vi "Cluster-typedefControls.vi"() -> ()   [LabVIEW 2016, in "test_ValueSignal.lvlib"]
uses:
  test_ValueSignal.lvlib
  main/apis/Stimulus/ValueSignalByPathString.vi
  main/apis/Assert/AssertControlValueByPathString.vi
  <vilib>/addons/_JKI Toolkits/Caraya/classes/Assert/Assert Equal Value and Type_Variant.vi
  <vilib>/addons/_JKI Toolkits/Caraya/classes/Test/Test.lvclass
  <vilib>/addons/_JKI Toolkits/Caraya/classes/Assert/Assert.lvclass
panel:
  out "error out":errorcluster
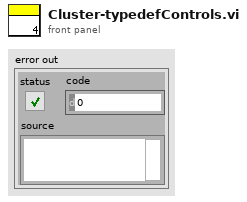
[diagram p1: front panel]
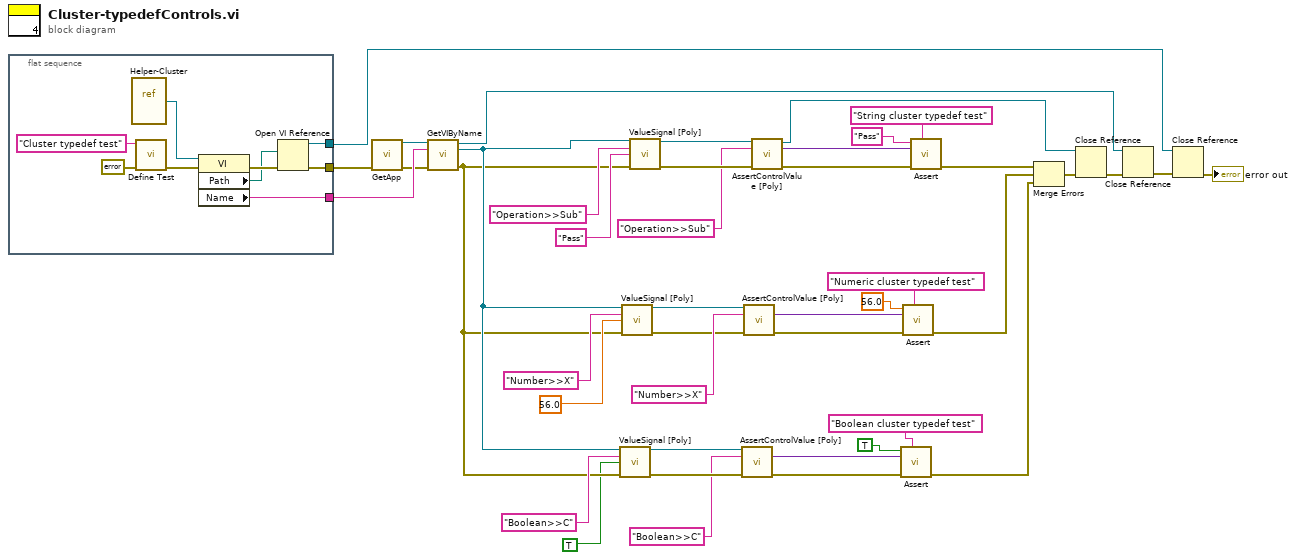
[diagram p0: block diagram]
diagram:
  n1 = flat-sequence {
    tunnel: [w48] -> w42
    tunnel: [w47] -> w27
    tunnel: [w45] -> w41
    frame #0 {
      n2 = vi-ref "Helper-Cluster.vi"() -> (w50:refnum<vi>)
      n3 = call <vilib>:"Define Test.vi"("error in (no error)"=errorcluster {"status"=FALSE, "code"=0, "source"=""}, "Label (VI Title)"="Cluster typedef test") -> ("error out"=w51:errorcluster)  [unwired: 9 in]
      n4 = property on="Property Node" class="VI"(reference=w50, error in=w51) -> (error out=w49:errorcluster, "Path"=w46:path, "Name"=w45:string)  [unwired: 1 out]
      n5 = Open VI Reference(vi path=w46, error in (no error)=w49) -> (vi reference=w47:refnum<vi>, error out=w48:errorcluster)  [unwired: 4 in]
    }
  }
  n6 = call "GetApp.vi"("error in (no error)"=w42) -> ("Application Ref"=w43:refnum<vi>, "error out"=w40:errorcluster)  [unwired: 13 in]
  n7 = call "GetVIByName.vi"("Application Ref in"=w43, "VI Name"=w41, "error in (no error)"=w40) -> ("Application Ref out"=w29:refnum<vi>, "VI Reference"=w5:refnum<vi>, "error out"=w4:errorcluster)  [unwired: 10 in]
  n8 = call-poly "ValueSignal [Poly].vi"("VI Reference In"=w5, "Control Name"="Boolean>>C", "Value (Signaling)"=TRUE, "error in"=w4) -> ("VI Reference Out"=w13:refnum<vi>, "error out"=w12:errorcluster)  [unwired: 10 in]
  n9 = call-poly "ValueSignal [Poly].vi"("VI Reference In"=w5, "Control Name"="Number>>X", "Value (Signaling)"=56.0, "error in"=w4) -> ("VI Reference Out"=w19:refnum<vi>, "error out"=w20:errorcluster)  [unwired: 10 in]
  n10 = call-poly "ValueSignal [Poly].vi"("VI Reference In"=w5, "Control Name"="Operation>>Sub", "Value (Signaling)"="Pass" ("Control Name"), "error in"=w4) -> ("VI Reference Out"=w39:refnum<vi>, "error out"=w38:errorcluster)  [unwired: 10 in]
  n11 = call-poly "AssertControlValue [Poly].vi"("VI Reference In"=w13, "Control Name"="Boolean>>C", "error in"=w12) -> ("Value"=w8:variant, "error out"=w9:errorcluster)  [unwired: 10 in, 1 out]
  n12 = call-poly "AssertControlValue [Poly].vi"("VI Reference In"=w19, "Control Name"="Number>>X", "error in"=w20) -> ("Value"=w24:variant, "error out"=w23:errorcluster)  [unwired: 10 in, 1 out]
  n13 = call-poly "AssertControlValue [Poly].vi"("VI Reference In"=w39, "Control Name"="Operation>>Sub", "error in"=w38) -> ("VI Reference Out"=w31:refnum<vi>, "Value"=w33:variant, "error out"=w34:errorcluster)  [unwired: 10 in]
  n14 = call-poly <vilib>:"Assert.vi"("Label"="Boolean cluster typedef test" ("Label (VI Title)"), "error in (no error)"=w9, "Y"=w8, "X"=TRUE) -> ("error out"=w6:errorcluster)  [unwired: 7 in]
  n15 = call-poly <vilib>:"Assert.vi"("Label"="Numeric cluster typedef test" ("Label (VI Title)"), "error in (no error)"=w23, "Y"=w24, "X"=56.0) -> ("error out"=w16:errorcluster)  [unwired: 7 in]
  n16 = call-poly <vilib>:"Assert.vi"("Label"="String cluster typedef test" ("Label (VI Title)"), "error in (no error)"=w34, "Y"=w33, "X"="Pass" ("Control Name")) -> ("error out"=w18:errorcluster)  [unwired: 7 in]
  n17 = Merge Errors(w18, w16, w6) -> (w17:errorcluster)
  n18 = Close Reference(reference=w31, error in (no error)=w17) -> (error out=w30:errorcluster)
  n19 = Close Reference(reference=w29, error in (no error)=w30) -> (error out=w28:errorcluster)
  n20 = Close Reference(reference=w27, error in (no error)=w28) -> (error out=→"error out":errorcluster)
